vi "ULx Acq&Graph Voltage-Int Clk.vi"() -> ()   [LabVIEW 2016]
doc: "I. Description:\nThis example demonstrates how to acquire a finite amount of data (waveform) using the DAQ device's internal clock.\n\nII. Instructions for Running:\n1. Select the physical channel to correspond to where your signal is input on the DAQ device.\n2. Enter the minimum and maximum voltages.\nNote: For better accuracy try to match the input range to the expected voltage level of the measured signal.\n3. Select the number of samples to acquire.\n4. Set the rate of the acquisition\nNote: The rate should be AT LEAST twice as fast as the maximum frequency component of the signal being acquired.\n\nIII. Block Diagram Steps:\n1. Create an analog input voltage channel.\n2. Set the rate for the sample clock. Additionally, define the sample mode to be finite and set the number of samples to be acquired per channel.\n3. Call the Start VI to start the acquisition.\n4. Use the Read VI to measure multiple samples from N Channels on the device. Set a timeout so an error is returned if the samples are not returned in the specified time limit\n5. Call the Clear Task VI to clear the Task.\n6. Use the popup dialog box to display an error if any.\n \nIV. I/O Connections Overview:\nMake sure your signal input terminal matches the Physical Channel I/O Control. For further connection information, refer to your hardware reference manual."
uses:
  <vilib>/Utility/error.llb/DialogType.ctl
  <vilib>/ULx/Create Channel.llb/ULx Create Channel (AI-Voltage-Basic).vi
  <vilib>/ULx/Timing.llb/ULx Timing (Sample Clock).vi
  <vilib>/ULx/Read.llb/ULx Read (Analog 1D Wfm NChan NSamp).vi
  <vilib>/measure/madcrms.llb/Basic Averaged DC-RMS for 1 Chan.vi
  <vilib>/measure/NI_MAPro.lvlib
panel:
  in  "Window Size":i32
  in  "Window Data":bool
  out "XY Graph":cluster{"Y":dbl[], "Y":dbl[]}[](graph)
  out "Time (s)":dbl
  out "Numeric":i32
  in  "stop":bool
  out "In Range?":bool
  out "Elapsed ms":u32
  in  "Channel Data Rate S/s":dbl=3720.0 format="%#_13g"
  out "Number of Channels":u16
  out "Acq Time (s)":dbl
  out "timeout":dbl=10.0 format="%0.2f"
  in  "Physical Channel":refnum<k21>="Dev0/Ai0"
  in  "Maximum Value":dbl=5.0 format="%0.2f"
  in  "Minimum Value":dbl=-5.0 format="%0.2f"
  out "Rate":dbl=1000.0 caption="Sample Rate (Hz)"
  in  "Samples per Channel":i32=1000
  out "Measurement":waveform(dbl)[](graph)
  # "For instructions, select Help>>Show Context Help"
  # "Channel Parameters"
  # "Timing Parameters"
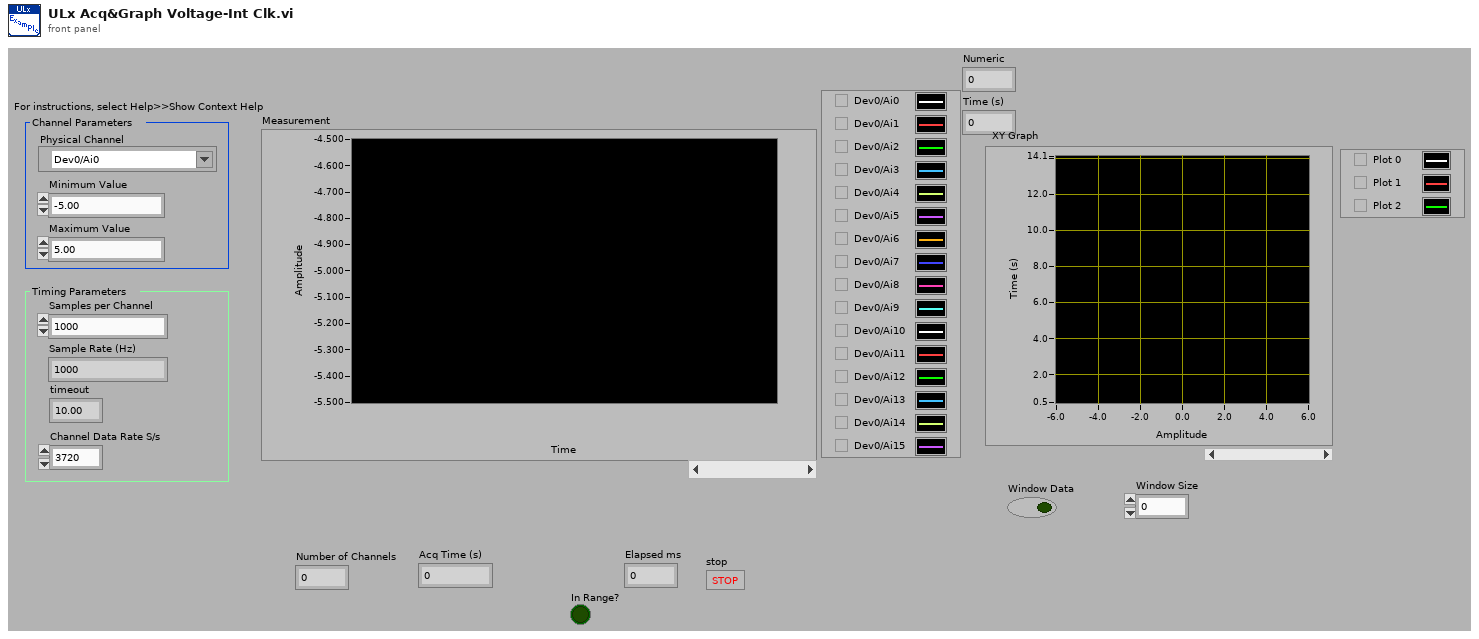
[diagram p1: front panel]
types:
  T1 = typedef "DialogType.ctl" = u16
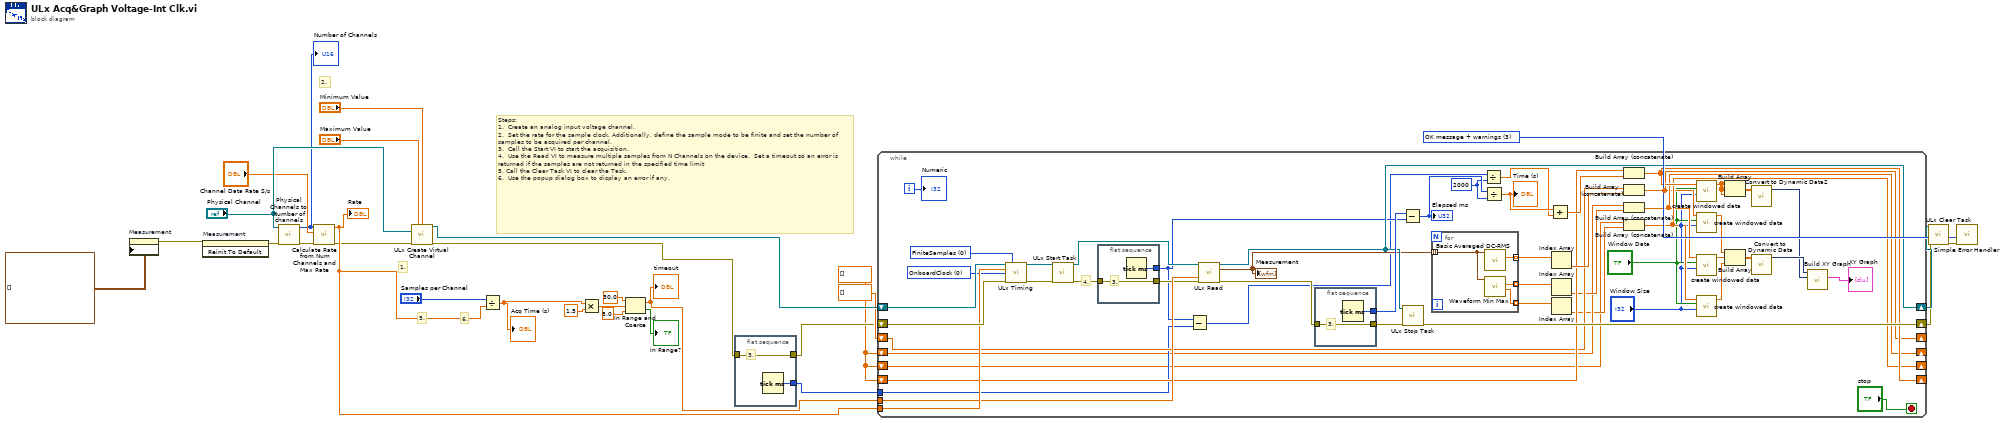
[diagram p0: block diagram]
diagram:
  w1 = dbl[] []
  w28 = T1 3 items=["no dialog", "OK message", "continue or stop message", "OK message + warnings", "continue/stop + warnings"] ("type of dialog (OK msg:1)")
  # "6."
  # "5."
  # "Steps: \n1.  Create an analog input voltage channel.\n2.  Set the rate for the sample clock. Additionally, define the sample mode to be finite and set the number of samples to be acquired per channel.\n3.  Call the Start VI to start the acquisition.\n4.  Use the Read VI to measure multiple samples from N Channels on the device.  Set a timeout so an error is returned if the samples are not returned in the specified time limit\n5. Call the Clear Task VI to clear the Task.\n6.  Use the popup dialog box to display an error if any."
  # "2."
  # "1."
  n1 = property on="Measurement" class="WFChart (strict)"("History Data"=waveform(dbl)[][] []) -> (error out=w7:errorcluster)  [unwired: 2 in, 1 out]
  n2 = invoke on="Measurement" class="WFChart (strict)" method="Reinit To Default"(error in=w7) -> (error out=w10:errorcluster)  [unwired: 2 in, 2 out]
  n3 = call "Physical Channels to Number of channels.vi"("error in (no error)"=w10, "Physical Channel in"="Physical Channel") -> ("error out"=w9:errorcluster, "Number of Channels"=w22:i32)  [unwired: 7 in, 1 out]
  "Number of Channels" <- w22
  n4 = call "Calculate Rate from Num Channels and Max Rate.vi"("error in (no error)"=w9, "Channel Data Rate S/s"="Channel Data Rate S/s", "Number of Channels"=w22) -> ("error out"=w8:errorcluster, "Rate"=w21:dbl)  [unwired: 7 in]
  "Rate" <- w21
  n5 = call-poly <vilib>:"ULx Create Virtual Channel.vi"("maximum value"="Maximum Value", "minimum value"="Minimum Value", "physical channels"="Physical Channel", "error in"=w8) -> ("task out"=w29:refnum<k24>, "error out"=w4:errorcluster)  [unwired: 10 in]
  n6 = Divide(x="Samples per Channel", y=w21) -> (x/y=w20:dbl)
  "Acq Time (s)" <- w20
  n7 = Multiply(x=w20, y=1.5) -> (x*y=w18:dbl)
  n8 = In Range and Coerce(upper limit=30.0, x=w18, lower limit=5.0) -> (coerced(x)=w15:dbl, In Range?=→"In Range?":bool)
  "timeout" <- w15
  n9 = flat-sequence {
    tunnel: [w31] -> w3
    tunnel: w4 -> [w31]
    tunnel: [w30] -> w2
    frame #0 {
      # "3."
      n10 = Tick Count (ms)() -> (millisecond timer value=w30:u32)
    }
  }
  n11 = while {
    tunnel: w21 -> [w80]
    tunnel: w15 -> [w79]
    shift-right: [w68] -> w12
    shift-left: w3 -> [w83]
    shift-right: [w67] -> w13
    shift-left: w29 -> [w82]
    shift-right: [w40] -> _
    shift-left: w1 -> [w55]
    shift-right: [w35] -> _
    shift-left: dbl[] [] -> [w54]
    tunnel: w2 -> [w52]
    shift-right: [w37] -> _
    shift-left: w1 -> [w49]
    shift-right: [w39] -> _
    shift-left: w1 -> [w46]
    i -> [w64]
    stop <- "stop" stop-if-true
    w58 = u32 2000 ("y")
    w70 = 0 items=["OnboardClock", "ExternalClock", "NoClock"] ("clock source")
    w71 = 0 items=["FiniteSamples", "ContinuousSamples"] ("sample mode")
    # "4."
    n12 = call-poly <vilib>:"ULx Timing.vi"("task in"=w82, "sample mode"=w71, "rate"=w80, "clock source"=w70, "error in"=w83) -> ("task out"=w81:refnum<k24>, "error out"=w76:errorcluster)  [unwired: 9 in]
    n13 = call <vilib>:"ULx Start Task.vi"("task in"=w81, "error in"=w76) -> ("task out"=w77:refnum<k24>, "error out"=w78:errorcluster)  [unwired: 12 in]
    n14 = flat-sequence {
      tunnel: [w89] -> w73
      tunnel: w78 -> [w89]
      tunnel: [w88] -> w59
      frame #0 {
        # "3."
        n15 = Tick Count (ms)() -> (millisecond timer value=w88:u32)
      }
    }
    n16 = Subtract(x=w59, y=w52) -> (x-y=w53:u32)
    n17 = call-poly <vilib>:"ULx Read.vi"("task in"=w77, "timeout"=w79, "error in"=w73) -> ("task out"=w67:refnum<k24>, "data"=w66:waveform(dbl)[], "error out"=w75:errorcluster)  [unwired: 10 in]
    "Measurement" <- w66
    n18 = flat-sequence {
      tunnel: [w91] -> w69
      tunnel: w75 -> [w91]
      tunnel: [w90] -> w74
      frame #0 {
        # "3."
        n19 = Tick Count (ms)() -> (millisecond timer value=w90:u32)
      }
    }
    n20 = Subtract(x=w74, y=w59) -> (x-y=w65:u32)
    "Elapsed ms" <- w65
    n21 = call <vilib>:"ULx Stop Task.vi"("error in"=w69, "task in"=w67) -> ("error out"=w68:errorcluster)  [unwired: 8 in, 1 out]
    n22 = for {
      tunnel: w66 -> [w86] mode=indexing
      tunnel: [w87] -> w62 mode=indexing
      tunnel: [w85] -> w50 mode=indexing
      tunnel: [w84] -> w48 mode=indexing
      n23 = call-poly <vilib>:"Basic Averaged DC-RMS.vi"("signal in"=w86) -> ("RMS value"=w87:dbl)  [unwired: 7 in, 3 out]
      n24 = call <vilib>:"Waveform Min Max.vi"("waveform in"=w86) -> ("Y min"=w84:dbl, "Y max"=w85:dbl)  [unwired: 5 in, 4 out]
    }
    n25 = Divide(x=w53, y=w58) -> (x/y=w60:dbl)
    n26 = Divide(x=w65, y=w58) -> (x/y=w63:dbl)
    "Time (s)" <- w63
    n27 = Add(x=w63, y=w60) -> (x+y=w61:dbl)
    n28 = Index Array(array=w62) -> (element=w57:dbl)  [unwired: 1 in]
    n29 = Index Array(array=w50) -> (element=w51:dbl)  [unwired: 1 in]
    n30 = Index Array(array=w48) -> (element=w47:dbl)  [unwired: 1 in]
    n31 = Build Array (concatenate)(w55, w61) -> (w40:dbl[])
    n32 = Build Array (concatenate)(w54, w57) -> (w35:dbl[])
    n33 = Build Array (concatenate)(w49, w51) -> (w37:dbl[])
    n34 = Build Array (concatenate)(w46, w47) -> (w39:dbl[])
    n35 = call "create windowed data.vi"("Window Size"="Window Size", "Window Data"="Window Data", "Array in"=w40) -> ("Array out"=w41:dbl[])  [unwired: 8 in]
    n36 = call "create windowed data.vi"("Window Size"="Window Size", "Window Data"="Window Data", "Array in"=w35) -> ("Array out"=w34:dbl[])  [unwired: 8 in]
    n37 = call "create windowed data.vi"("Window Size"="Window Size", "Window Data"="Window Data", "Array in"=w37) -> ("Array out"=w36:dbl[])  [unwired: 8 in]
    n38 = call "create windowed data.vi"("Window Size"="Window Size", "Window Data"="Window Data", "Array in"=w39) -> ("Array out"=w38:dbl[])  [unwired: 8 in]
    n39 = Build Array(w41, w41, w41) -> (w43:dbl[][])
    n40 = Build Array(w34, w36, w38) -> (w45:dbl[][])
    n41 = call "Convert to Dynamic Data2"("2D Array"=w43) -> ("Dynamic Data Type"=w42:dynamicdata)  [unwired: 3 in]
    n42 = call "Convert to Dynamic Data"("2D Array"=w45) -> ("Dynamic Data Type"=w44:dynamicdata)  [unwired: 3 in]
    n43 = call "Build XY Graph"("Y Input"=w42, "X Input"=w44) -> ("XY Graph"=→"XY Graph":cluster{"X":dbl[], "Y":dbl[]}[])  [unwired: 8 in, 1 out]
    "Numeric" <- w64
  }
  n44 = call <vilib>:"ULx Clear Task.vi"("task in"=w13, "error in"=w12) -> ("error out"=w11:errorcluster)  [unwired: 13 in]
  n45 = call <vilib>:"Simple Error Handler.vi"("type of dialog (OK msg:1)"=w28, "error in (no error)"=w11) -> ()  [unwired: 3 in, 5 out]
